vi "mediaBalls_v2.vi"(11 "Array Ball Pose + CamID":cluster{"x":sgl, "y":sgl, "camera_id":u32}[](array[cluster])) -> (3 "Ball out":cluster{"x":dbl, "y":dbl})   [LabVIEW 2018]
panel:
  in  "cluster":cluster{"x":dbl, "y":dbl}
  in  "Field Size 2":T1
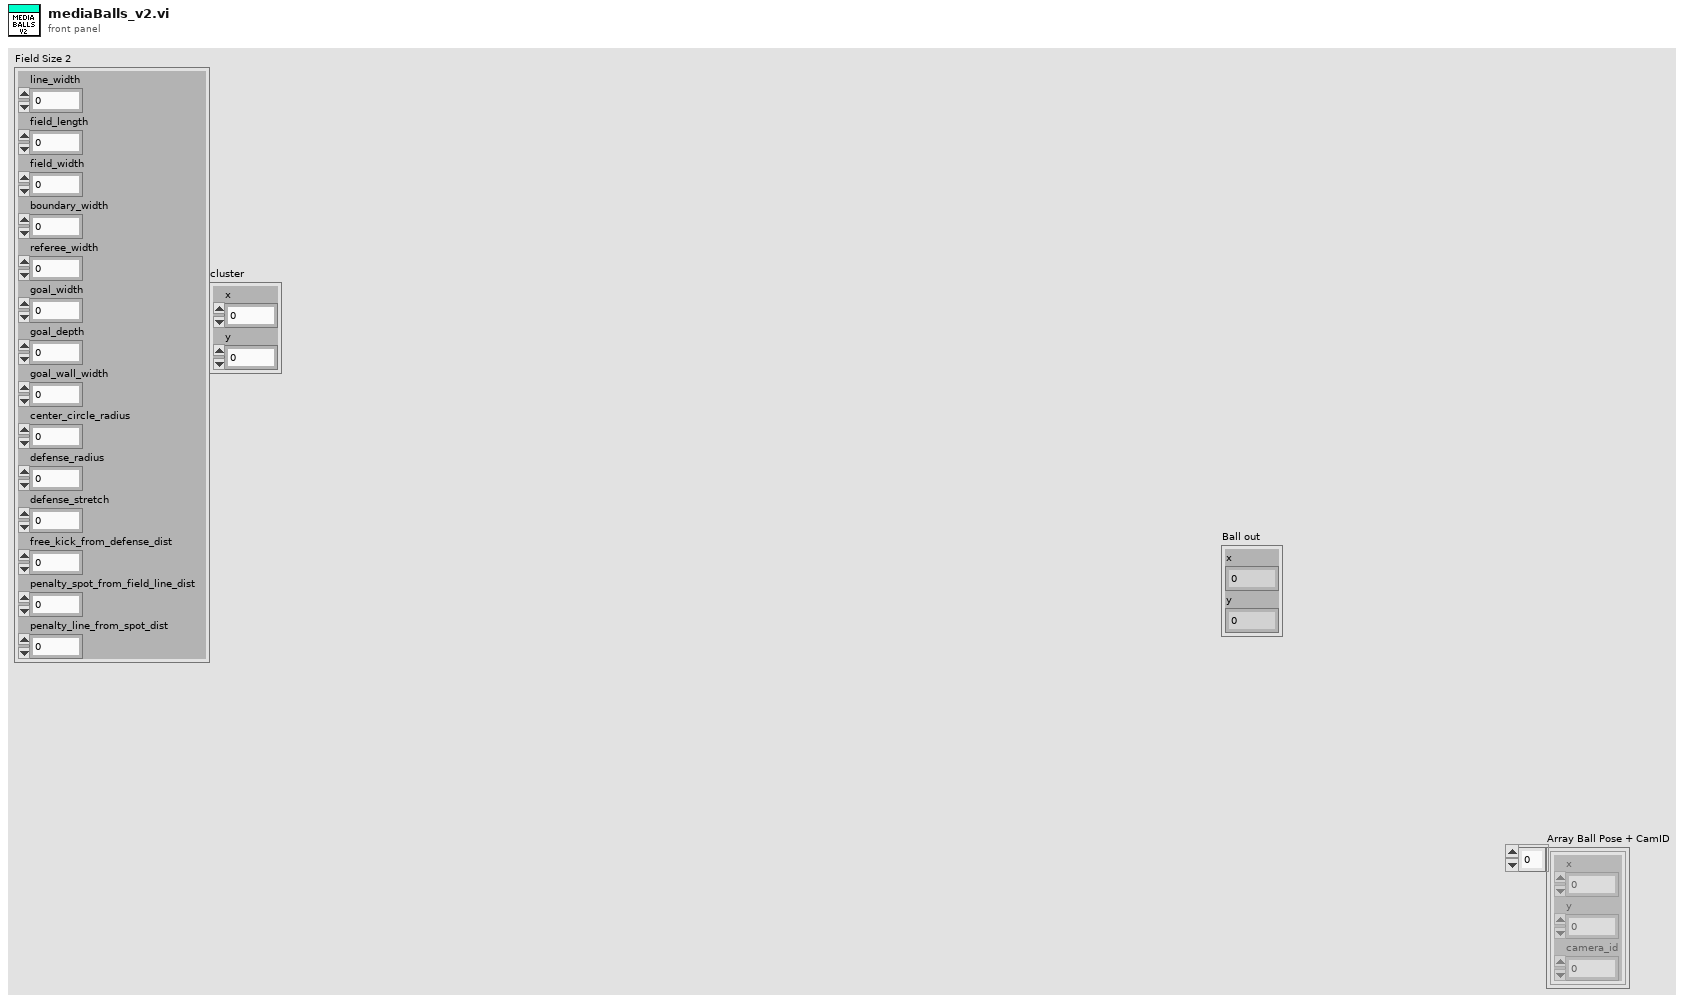
[diagram p1: front panel]
types:
  T1 = cluster{"line_width":u32, "field_length":u32, "field_width":u32, "boundary_width":u32, "referee_width":u32, "goal_width":u32, "goal_depth":u32, "goal_wall_width":u32, "center_circle_radius":u32, "defense_radius":u32, "defense_stretch":u32, "free_kick_from_defense_dist":u32, "penalty_spot_from_field_line_dist":u32, "penalty_line_from_spot_dist":u32}
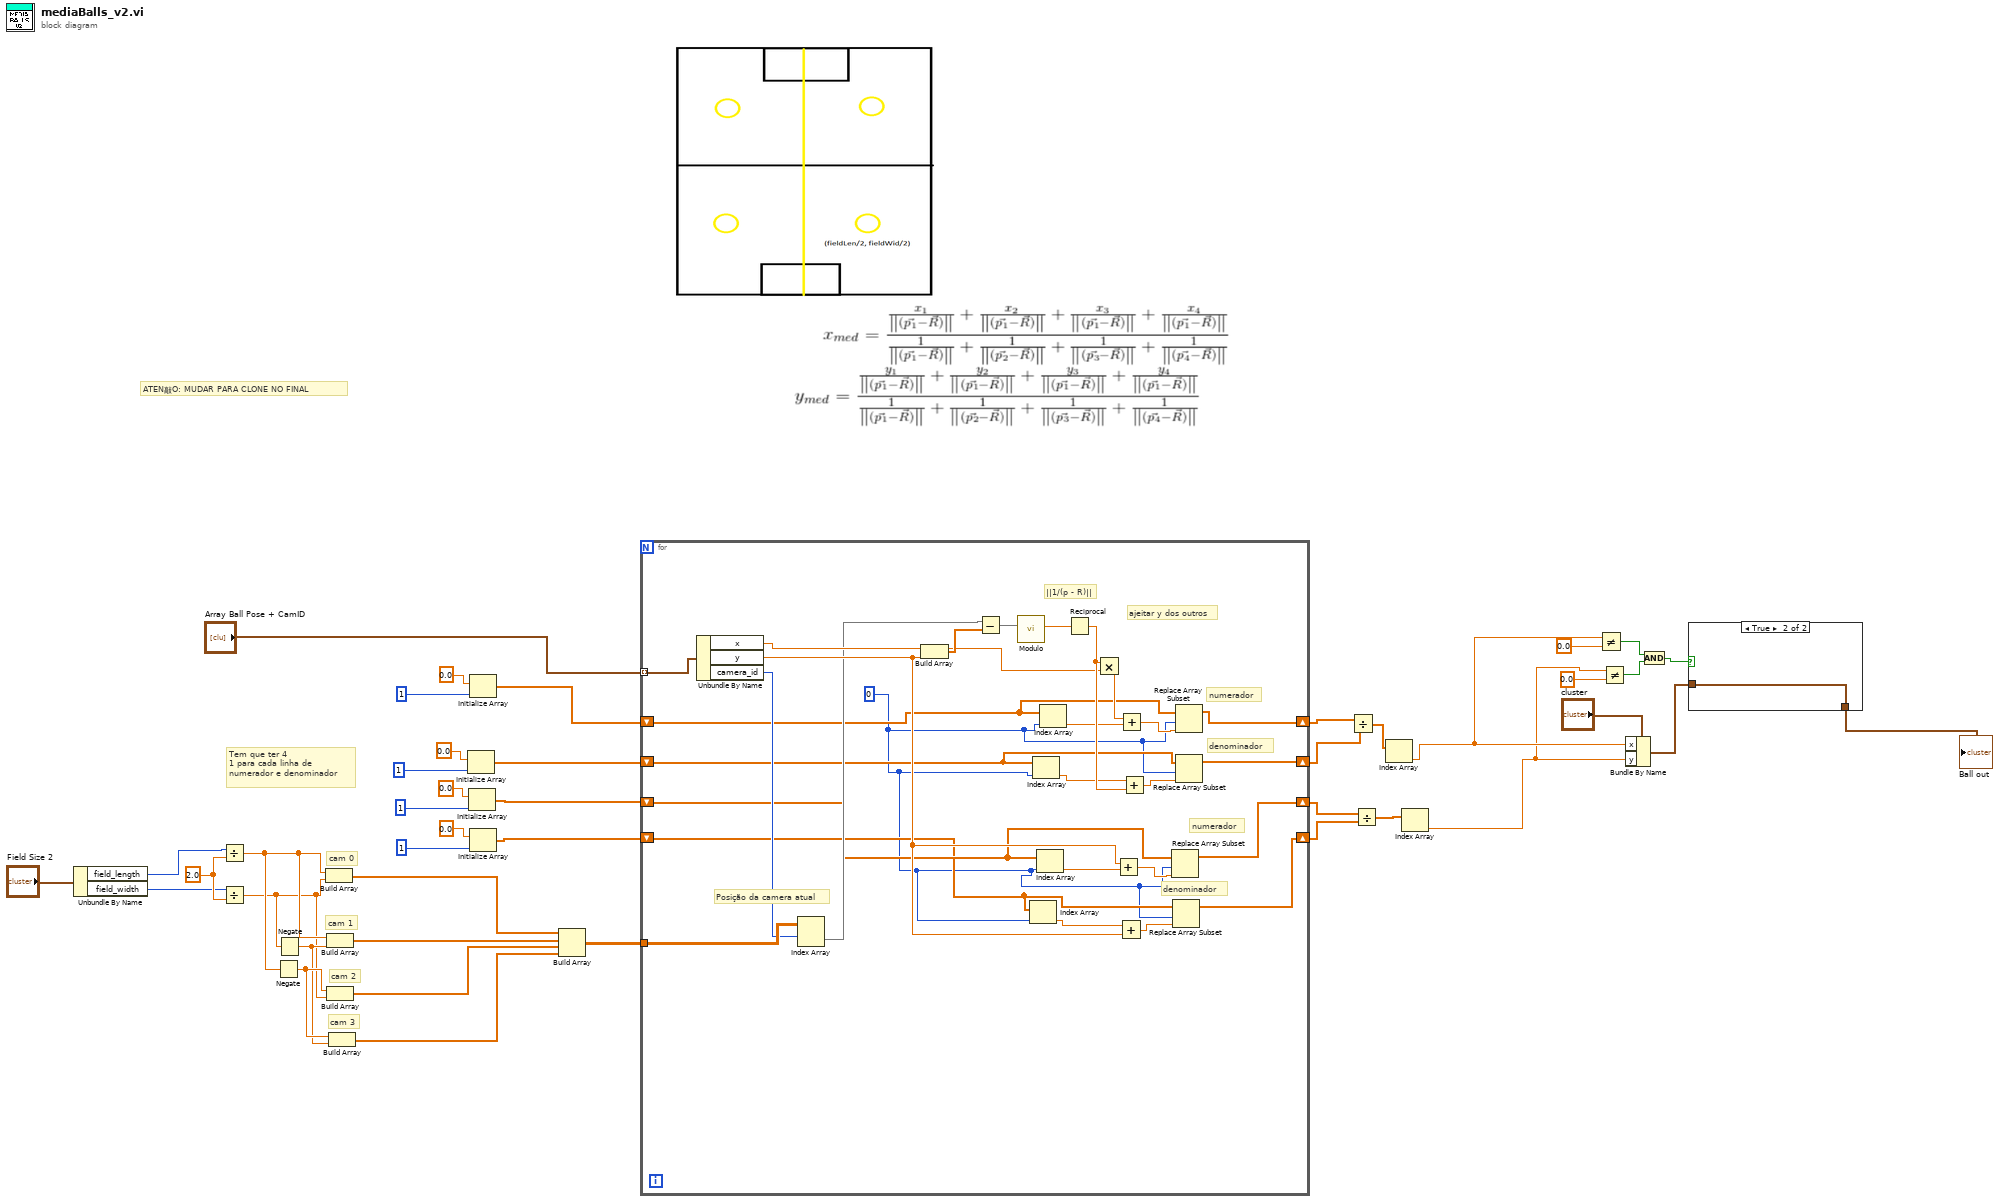
[diagram p0: block diagram]
diagram:
  w41 = 2.0 ("y")
  # "Tem que ter 4\n1 para cada linha de\nnumerador e denominador"
  # "cam 3"
  # "cam 2"
  # "cam 1"
  # "cam 0"
  # "ATEN敲O: MUDAR PARA CLONE NO FINAL"
  n1 = Unbundle By Name("Field Size 2") -> ("field_length"=w40:u32, "field_width"=w39:u32)
  n2 = Divide(x=w40, y=w41) -> (x/y=w37:dbl)
  n3 = Divide(x=w39, y=w41) -> (x/y=w35:dbl)
  n4 = Negate(x=w37) -> (-x=w38:dbl)
  n5 = Negate(x=w35) -> (-x=w36:dbl)
  n6 = Build Array(w37, w35) -> (w34:dbl[])
  n7 = Build Array(w37, w36) -> (w33:dbl[])
  n8 = Build Array(w38, w35) -> (w32:dbl[])
  n9 = Build Array(w38, w36) -> (w31:dbl[])
  n10 = Initialize Array(0.0 ("element"), 1 ("dimension size")) -> (w20:dbl[])
  n11 = Initialize Array(0.0 ("element"), 1 ("dimension size")) -> (w19:dbl[])
  n12 = Initialize Array(0.0 ("element"), 1 ("dimension size")) -> (w21:dbl[])
  n13 = Initialize Array(0.0 ("element"), 1 ("dimension size")) -> (w18:dbl[])
  n14 = Build Array(w34, w33, w32, w31) -> (w30:dbl[][])
  n15 = for {
    tunnel: "Array Ball Pose + CamID" -> [w70] mode=indexing
    tunnel: w30 -> [w69]
    shift-right: [w51] -> w17
    shift-left: w21 -> [w45]
    shift-right: [w50] -> w16
    shift-left: w20 -> [w44]
    shift-right: [w49] -> w15
    shift-left: w19 -> [w47]
    shift-right: [w48] -> w14
    shift-left: w18 -> [w46]
    w43 = 0 ("index")
    # "ajeitar y dos outros"
    # "denominador"
    # "numerador"
    # "denominador"
    # "numerador"
    # "||1/(p - R)||"
    # "Posição da camera atual"
    n16 = Unbundle By Name(w70) -> ("x"=w58:sgl, "y"=w57:sgl, "camera_id"=w68:u32)
    n17 = Index Array(array=w69, index (row)=w68) -> (element=w56:dbl[])  [unwired: 1 in]
    n18 = Build Array(w58, w57) -> (w67:sgl[])
    n19 = Subtract(x=w56, y=w67) -> (x-y=w66:dbl[])
    n20 = call "Modulo.vi"("2D vector"=w66) -> ("Modulo"=w65:dbl)  [unwired: 10 in]
    n21 = Index Array(array=w46, index=w43) -> (element=w52:dbl)
    n22 = Index Array(array=w44, index=w43) -> (element=w54:dbl)
    n23 = Index Array(array=w47, index=w43) -> (element=w53:dbl)
    n24 = Index Array(array=w45, index=w43) -> (element=w55:dbl)
    n25 = Reciprocal(x=w65) -> (1/x=w59:dbl)
    n26 = Multiply(x=w59, y=w58) -> (x*y=w64:dbl)
    n27 = Add(x=w57, y=w53) -> (x+y=w61:dbl)
    n28 = Add(x=w52, y=w57) -> (x+y=w60:dbl)
    n29 = Add(x=w64, y=w55) -> (x+y=w63:dbl)
    n30 = Add(x=w54, y=w59) -> (x+y=w62:dbl)
    n31 = Replace Array Subset(array=w47, new element=w61, index=w43) -> (w49:dbl[])
    n32 = Replace Array Subset(array=w46, new element=w60, index=w43) -> (w48:dbl[])
    n33 = Replace Array Subset(array=w45, new element=w63, index=w43) -> (w51:dbl[])
    n34 = Replace Array Subset(array=w44, new element=w62, index=w43) -> (w50:dbl[])
  }
  n35 = Divide(x=w17, y=w16) -> (x/y=w5:dbl[])
  n36 = Divide(x=w15, y=w14) -> (x/y=w3:dbl[])
  n37 = Index Array(array=w5) -> (element=w4:dbl)  [unwired: 1 in]
  n38 = Index Array(array=w3) -> (element=w2:dbl)  [unwired: 1 in]
  n39 = Not Equal?(x=w4, y=0.0) -> (x != y?=w10:bool)
  n40 = Not Equal?(x=w2, y=0.0) -> (x != y?=w9:bool)
  n41 = Bundle By Name(cluster="cluster", "x"=w4, "y"=w2) -> (w7:cluster{"x":dbl, "y":dbl})
  n42 = And(x=w10, y=w9) -> (x .and. y?=w8:bool)
  n43 = case shown="True" w8 {
    tunnel: [w71 w72] -> w1
    tunnel: w7 -> [w71 w72]
    frame False {
    }
    frame True {
    }
  }
  "Ball out" <- w1
